vi "相机4结束录制视频.vi"(7 "Image Out":T1, 8 "Cam4队列":refnum<queue>, 9 "录视频开始时间":u32, 10 "锁附监控-开始录视频":bool, 11 "引用句柄输入":T2) -> (0 "录制时间":u32, 3 "视频录制中":bool)   [LabVIEW 2014]
uses:
  <vilib>/vision/Avi.llb/IMAQ AVI2 Refnum.ctl
  <vilib>/vision/Image Controls.llb/IMAQ Image.ctl
  Controls/Cam4QueueAction.ctl
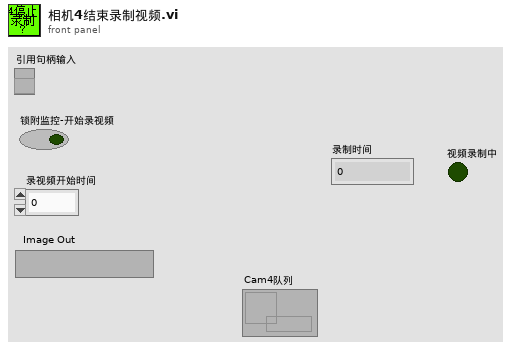
[diagram p1: front panel]
types:
  T1 = typedef "IMAQ Image.ctl" = refnum<image>
  T2 = typedef "IMAQ AVI2 Refnum.ctl" = refnum<k20>
  T3 = typedef "Cam4QueueAction.ctl" = enum16{"Cam4初始化", "Cam4更新曝光时间", "Cam4等待", "Cam4实时", "Cam4录视频初始化", "Cam4结束录视频"}
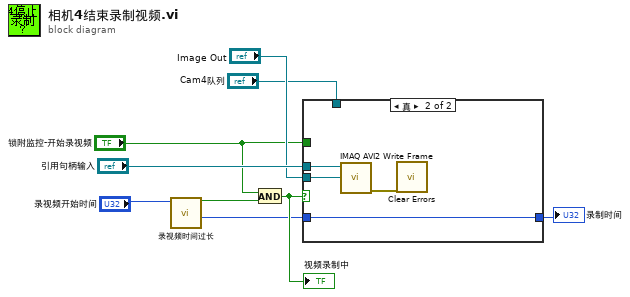
[diagram p0: block diagram]
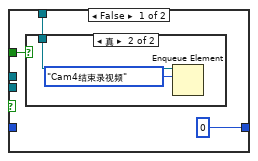
[diagram p2: hidden frame]
diagram:
  n1 = call "录视频时间过长.vi"("录视频初始时间"="录视频开始时间") -> ("录制时间"=w3:u32, "录制时间在规格内"=w8:bool)  [unwired: 9 in]
  n2 = And(x="锁附监控-开始录视频", y=w8) -> (x .and. y?=w9:bool)
  "视频录制中" <- w9
  n3 = case shown="真" w9 {
    tunnel: "引用句柄输入" -> [_ w18]
    tunnel: "Image Out" -> [_ w17]
    tunnel: "Cam4队列" -> [w12 _]
    tunnel: w3 -> [_ w15]
    tunnel: [u32 0 ("录制时间") w15] -> w2
    tunnel: "锁附监控-开始录视频" -> [w10 _]
    frame False {
      n4 = case shown="真" w10 {
        tunnel: w12 -> [_ w14]
        frame False {
        }
        frame True {
          n5 = Enqueue Element(queue=w14, element=Cam4QueueAction."Cam4结束录视频" ("元素")) -> ()  [unwired: 2 in, 3 out]
        }
      }
    }
    frame True {
      n6 = call "IMAQ AVI2 Write Frame"("Image"=w17, "AVI Refnum"=w18) -> ("error out"=w16:errorcluster)  [unwired: 7 in, 2 out]
      n7 = call <vilib>:"Clear Errors.vi"("error in (no error)"=w16) -> ()  [unwired: 5 in, 2 out]
    }
  }
  "录制时间" <- w2
